vi "Read Replicated.vi"(8 "error in (no error)":errorcluster, 11 "third in":refnum<class "third.lvclass">) -> (0 "error out":errorcluster, 2 "Replicated":bool, 3 "third out":refnum<class "third.lvclass">)   [LabVIEW 2015, in "third.lvclass"]
uses:
  third.lvclass
  third.lvclass/third.ctl
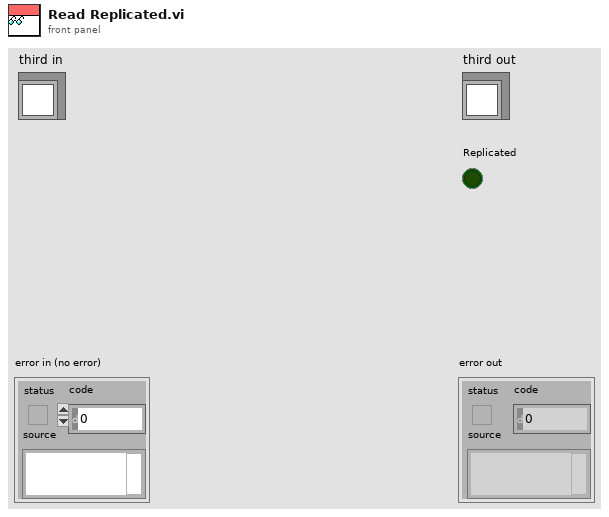
[diagram p1: front panel]
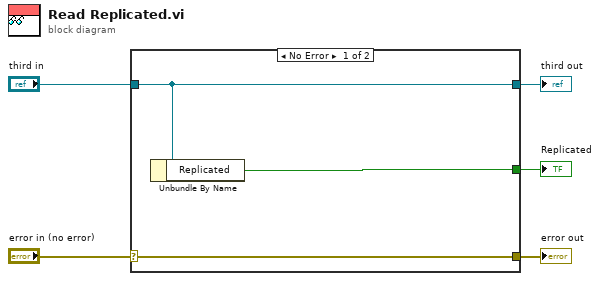
[diagram p0: block diagram]
diagram:
  n1 = case shown="No Error" "error in (no error)" {
    selector: "error in (no error)" -> [w8 w9]
    tunnel: [w8 w9] -> w4
    tunnel: [w7 w10] -> w2
    tunnel: "third in" -> [w7 w10]
    tunnel: [w6 _] -> w1
    frame No Error {
      n2 = Unbundle By Name(w7) -> ("Replicated"=w6:bool)
    }
    frame Error {
    }
  }
  "error out" <- w4
  "third out" <- w2
  "Replicated" <- w1
